vi "DetectBarcodesGreyscale.vi"(8 "error in (no error)":errorcluster, 10 "Greyscale Image":refnum<data-value>, 11 "BarcodeDetector in":refnum<class "BarcodeDetector.lvclass">) -> (0 "error out":errorcluster, 2 "Detections":T1[](array[typedef]), 3 "BarcodeDetector (Duplicate)":refnum<class "BarcodeDetector.lvclass">)   [LabVIEW 2020, in "g_ar_toolkit.feature_detection.lvlib" / "BarcodeDetector.lvclass"]
uses:
  BarcodeDetector.lvclass
  Detection.ctl
  Detection Region.ctl
  g_ar_toolkit.common/Image Point (Integer).ctl
  BarcodeDetector.lvclass/BarcodeDetector.ctl
  g_ar_toolkit.common/Module Path.vi
  <vilib>/Utility/error.llb/Error Cluster From Error Code.vi
  ed9d7ada-6e4f-470f-8132-b218d1fc92ad.vi
  g_ar_toolkit.common/g_ar_toolkit.common.lvlib
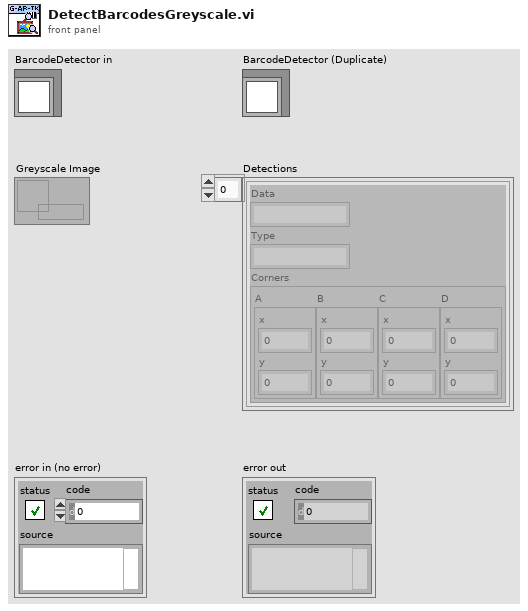
[diagram p1: front panel]
types:
  T1 = typedef "g_ar_toolkit.feature_detection.lvlib/BarcodeDetector.lvclass/Detection.ctl" = cluster{"Data":string, "Type":string, "Corners":T2}
  T2 = typedef "g_ar_toolkit.feature_detection.lvlib/BarcodeDetector.lvclass/Detection Region.ctl" = cluster{"A":T3, "B":T3, "C":T3, "D":T3}
  T3 = typedef "g_ar_toolkit.common.lvlib/Image Point (Integer).ctl" = cluster{"x":i32, "y":i32}
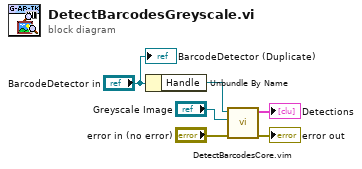
[diagram p0: block diagram]
diagram:
  n1 = Unbundle By Name("BarcodeDetector in") -> ("Handle"=w1:refnum<data-value>)
  n2 = call "DetectBarcodesCore.vim"("error in (no error)"="error in (no error)", "Greyscale Image"="Greyscale Image", "Handle"=w1) -> ("error out"=→"error out":errorcluster, "Detections"=→"Detections":T1[])  [unwired: 7 in]
  "BarcodeDetector (Duplicate)" <- "BarcodeDetector in"
